vi "LS336 Heater Range.vi"(0 "Heater Range":enum16{"OFF", "LOW", "MEIDUM", "HIGH"}(ring), 1 "Loop":bool, 2 "Lakeshore GPIB Address":refnum<visa-resource-name>) -> ()   [LabVIEW 2019]
panel:
  out "resulting string":string
  # "Which Heater to control?"
  # "Loop 2\n(Probe / 3He Pot)"
  # "Heater Range"
  # "Loop 1\n(Sorb / VTI)"
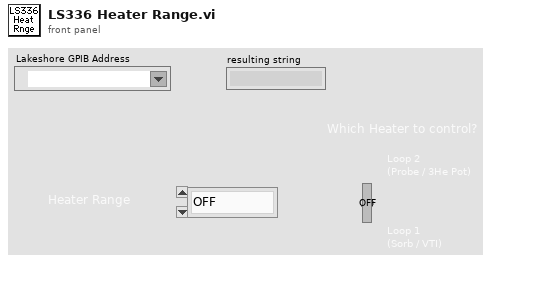
[diagram p1: front panel]
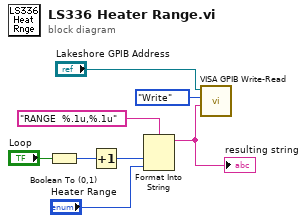
[diagram p0: block diagram]
diagram:
  n1 = Boolean To (0,1)(Boolean="Loop") -> (0, 1=w3:i16)
  n2 = Increment(x=w3) -> (x+1=w2:i16)
  n3 = Format Into String(format string="RANGE  %.1u,%.1u" ("initial string"), w2, "Heater Range") -> (resulting string=w6:string)  [unwired: 2 in, 1 out]
  "resulting string" <- w6
  n4 = call "VISA GPIB Write-Read.vi"("Command"=w6, "Action"=enum16{"Write", "Read", "Write & Read"}."Write", "VISA resource name"="Lakeshore GPIB Address") -> ()  [unwired: 5 in, 4 out]
